vi "connect Pdc.vi"(7 "pseudoPdcId":i32, 9 "pdcId":i32, 10 "port":i32, 11 "ipAddress":string) -> (2 "function return":i32, 3 "ipAddress out":string, 5 "pseudoPdcId out":i32)   [LabVIEW 2018, in "S3DK.lvlib" / "C37118-DLL.lvlib" / "StrongridDLL.lvlib"]
doc: "STRONGRIDIEEEC37118DLL_API int __cdecl connectPdc( char *ipAddress, int port, int32_t pdcId, int32_t* pseudoPdcId);"
uses:
  StrongridDLL.lvlib
  <vilib>/builds/S3DK Compiler/My Packed Library/StrongridDLL.dll
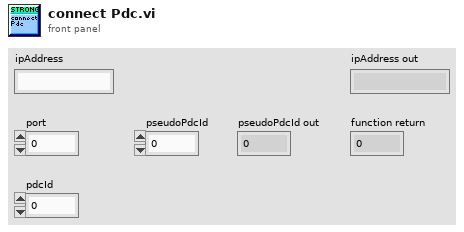
[diagram p1: front panel]
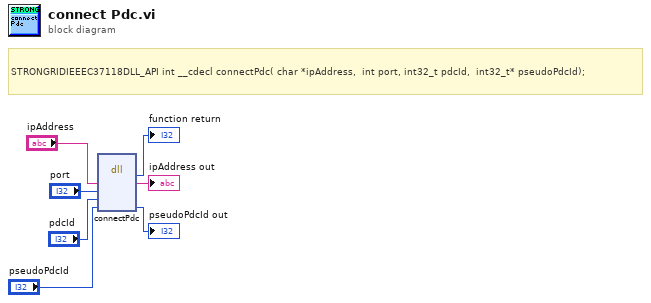
[diagram p0: block diagram]
diagram:
  # "STRONGRIDIEEEC37118DLL_API int __cdecl connectPdc( char *ipAddress,  int port, int32_t pdcId,  int32_t* pseudoPdcId);"
  n1 = dll-call lib="C:/Program Files/National Instruments/LabVIEW 2018/vi.lib/builds/S3DK Compiler/My Packed Library/StrongridDLL.dll" fn="connectPdc"("ipAddress"="ipAddress", "port"="port", "pdcId"="pdcId", "pseudoPdcId"="pseudoPdcId") -> ("return type"=→"function return":i32, "ipAddress"=→"ipAddress out":string, "pseudoPdcId"=→"pseudoPdcId out":i32)  [unwired: 5 in, 2 out]
